vi "Actor Core.vi"(8 "error in":errorcluster, 11 "WebServer in":refnum<class "MonSys_Server_Actor.lvclass">) -> (0 "error out":errorcluster, 3 "Actor out":refnum<class "Actor.lvclass">)   [LabVIEW 2018, in "MonSys_Server_Actor.lvlib" / "MonSys_Server_Actor.lvclass"]
doc: "(<B>Filename</B>: Actor Framework.lvlib:Actor.lvclass:Actor Core.vi)\n\nReceives messages to the actor, reacts to them, and initiates any error handling that may shut the actor down.\n\nDescendant classes may override this VI to append parallel tasks for the actor to complete while it handles messages. Overrides use the Call Parent Method node."
uses:
  MonSys_Server_Actor.lvclass
  <vilib>/ActorFramework/Actor/Actor.lvclass
  MonSys_Server_Actor.lvclass/MonSys_Server_Actor.ctl
  typedefs/OnlineData_HandleDVR_func.ctl
  <extravilib>/ChannelInstances/Tag-bool/Read With Abort.vi
  <extravilib>/ChannelInstances/Tag-bool/Write With Abort.vi
  <extravilib>/ChannelInstances/Tag-bool/Instantiate.vi
  <extravilib>/ChannelInstances/Tag-bool/EndpointRead.vi
  WebResources/GLB_WebService_Status.vi
  <extravilib>/ChannelInstances/Tag-bool/Endpoint.vi
  <extravilib>/ChannelInstances/Tag-bool.lvlib
panel:
  out "Computer Name":string
  out "Web Service Status":bool
  out "Local IP Address":string
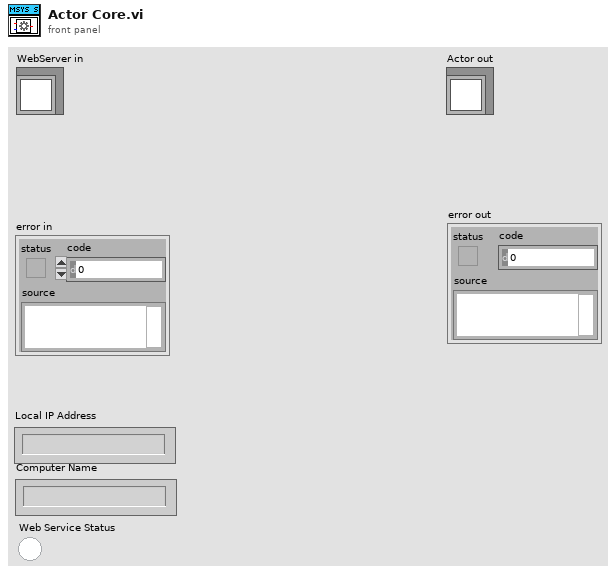
[diagram p1: front panel]
types:
  T1 = enum32{"Invalid", "Standard", "Closed", "Hidden", "Minimized", "Maximized"}
  T2 = typedef "OnlineData_HandleDVR_func.ctl" = enum16{"create", "get", "close"}
  T3 = typedef "Tag-bool.lvlib/))Channel.ctl" = refnum<queue>
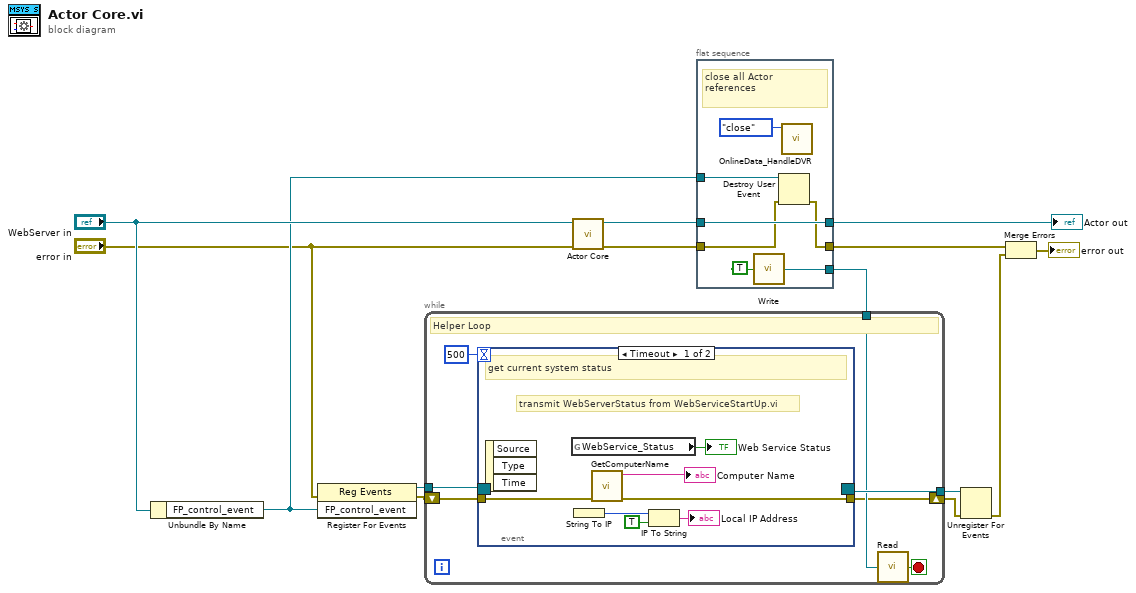
[diagram p0: block diagram]
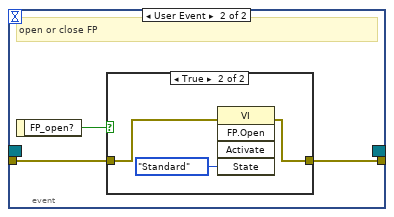
[diagram p2: hidden frame]
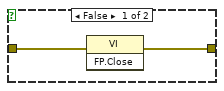
[diagram p3: hidden frame]
diagram:
  n1 = Unbundle By Name("WebServer in") -> ("FP_control_event"=w11:refnum<user-event>)
  n2 = register-events(error in="error in", w11) -> (reference out=w10:refnum<event-registration>, error out=w3:errorcluster)  [unwired: 1 in]
  n3 = while {
    tunnel: w10 -> [w21]
    tunnel: [w20] -> w9
    tunnel: w8 -> [w19]
    shift-right: [w16] -> w2
    shift-left: w3 -> [w17]
    stop <- w18 stop-if-true
    # "Helper Loop"
    n4 = event shown="[0] Timeout" {
      selector: w21 -> [_ _]
      dyn-events: [_ _] -> w20
      timeout: 500 -> [_ _]
      tunnel: w17 -> [w24 w30]
      tunnel: [w23 w29] -> w16
      event Timeout {
        # "transmit WebServerStatus from WebServiceStartUp.vi"
        # "get current system status"
        n5 = event-data() -> ()  [unwired: 1 in, 3 out]
        n6 = global read "GLB_WebService_Status.vi" "WebService_Status"() -> (→"Web Service Status":bool)
        n7 = String To IP() -> (0:w28:u32)  [unwired: 1 in]
        n8 = call "GetComputerName.vi"("error in (no error)"=w24) -> ("error out"=w23:errorcluster, "lpbuffer (Computer Name)"=→"Computer Name":string)  [unwired: 9 in]
        n9 = IP To String(1:TRUE ("dot notation? (F)"), 2:w28) -> (0:→"Local IP Address":string)
      }
      event User Event {
        # "open or close FP"
        n10 = event-data() -> ("FP_open?"=w31:bool)  [unwired: 1 in]
        n11 = case shown="True" w31 {
          tunnel: w30 -> [w33 w34]
          tunnel: [w32 w35] -> w29
          frame False {
            n12 = invoke class="VI" method="FP.Close"(error in=w33) -> (error out=w32:errorcluster)  [unwired: 2 in, 2 out]
          }
          frame True {
            n13 = invoke class="VI" method="FP.Open"(error in=w34, "State"=T1."Standard") -> (error out=w35:errorcluster)  [unwired: 3 in, 4 out]
          }
        }
      }
    }
    n14 = call <extravilib>:"Read.vi"("channel"=w19) -> ("element"=w18:bool)  [unwired: 1 in, 1 out]
  }
  n15 = call-parent "Actor Core.vi"("error in"="error in", "Actor in"="WebServer in") -> ("error out"=w13:errorcluster, "Actor out"=w5:refnum<class "Actor.lvclass">)  [unwired: 8 in]
  n16 = flat-sequence {
    tunnel: [w37] -> w14
    tunnel: w13 -> [w38]
    tunnel: w11 -> [w42]
    tunnel: [w40] -> w8
    tunnel: w5 -> [w39]
    tunnel: [w39] -> w4
    frame #0 {
      # "close all Actor references"
      n17 = call <extravilib>:"Write.vi"("element"=TRUE ("Stop Button")) -> ("channel"=w40:T3)  [unwired: 1 out]
      n18 = Destroy User Event(user event=w42, error in=w38) -> (error out=w37:errorcluster)
      n19 = call "OnlineData_HandleDVR.vi"("func"=OnlineData_HandleDVR_func."close") -> ()  [unwired: 9 in, 2 out]
    }
  }
  n20 = Unregister For Events(event registration refnum=w9, error in=w2) -> (error out=w6:errorcluster)
  n21 = Merge Errors(w14, w6) -> (→"error out":errorcluster)
  "Actor out" <- w4
